vi "Control Model to Model of operation.vi"(1 "Control Mode":u8(ring)=2 items=["Velocity"=2, "Torque"=1]) -> (0 "Mode of operation":i8(ring)=9 items=["Induction VF – testing purposes only"=-5, "Aligning rotor position"=-4, "Current stepper – testing purposes only "=-3, "Voltage stepper – testing purposes only"=-2, "Voltage constant angle – testing purposes only"=-1, "No mode"=0, "Cyclic sync position"=8, "Cyclic sync velocity"=9, "Cyclic sync torque"=10])   [LabVIEW 2016]
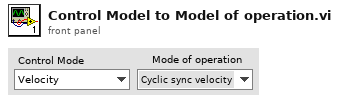
[diagram p1: front panel]
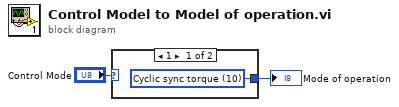
[diagram p0: block diagram]
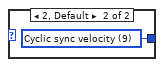
[diagram p2: hidden frame]
diagram:
  n1 = case shown="1" "Control Mode" {
    tunnel: [w3 w4] -> w1
    frame 1 {
      w3 = i8 10 items=["Induction VF – testing purposes only"=-5, "Aligning rotor position"=-4, "Current stepper – testing purposes only "=-3, "Voltage stepper – testing purposes only"=-2, "Voltage constant angle – testing purposes only"=-1, "No mode"=0, "Cyclic sync position"=8, "Cyclic sync velocity"=9, "Cyclic sync torque"=10] ("Mode of operation")
    }
    frame 2, Default {
      w4 = i8 9 items=["Induction VF – testing purposes only"=-5, "Aligning rotor position"=-4, "Current stepper – testing purposes only "=-3, "Voltage stepper – testing purposes only"=-2, "Voltage constant angle – testing purposes only"=-1, "No mode"=0, "Cyclic sync position"=8, "Cyclic sync velocity"=9, "Cyclic sync torque"=10] ("Mode of operation")
    }
  }
  "Mode of operation" <- w1
